vi "Compressor With Cylinder.vi"() -> ()   [LabVIEW 2014]
doc: "Compressor with Cylinder \n\nThis example shows how to control a compressor, extend and retract a cylinder, and optionally use a limit switch to retract automatically.\n\nThis example works with the PCM (Pneumatic Control Module) communicating with the roboRIO over CAN bus. The PCM must also be supplied with 12V DC from the PDP (Power Distribution Panel).\n\nThe Compressor, Pressure Switch, and Solenoids are all wired to the PCM \n\nThe Limit Switch is wired to DIO 9. It causes the cylinder to retract when the Auto Retract button is pressed.\n\nRefer to the Pneumatics Manual for air connections. Your pneumatics setup should include a compressor, pressure switch, tank, regulator, valve, flow controls, cylinder, plug valve, etc.\n\nTo run this example you should have a pneumatic system with air pressure connected to the P input on the SMC double solenoid valve. The A output of the valve should be connected via a flow control to the backend of a cylinder. The B output of the valve should be connected via a flow control to the frontend of a cylinder. When the cylinder is extended, it should physically depress the Limit Switch.\n\nWith the VI running, pressing the Extend button will push the cylinder shaft out, and pressing the Retract button will pull it back. Notice that the Extend and Retract buttons have their Mechanical Action set to Latch When Pressed. This means they stay pressed (ON) until they are read by the program, then they return to the OFF position. This works because once the SMC solenoid valve is pulled one direction, it stays in that position until it is pulled in the opposite direction - it only needs to be momentarily energized. The Auto Retract button can be used to make the cylinder return automatically. With the Auto Retract button ON, pressing the Extend button will push the cylinder out, and it will retract when it hits the limit switch.\n\nThis example expects a USB cable connected from your development PC to the Type B USB Jack (next to the power input) on the roboRIO.\n\nThis example expects the Driver Station to be running."
uses:
  <vilib>/Rock Robotics/WPI/Solenoid/WPI_SolenoidChannel.ctl
  <vilib>/Rock Robotics/SystemInterfaces/DIO/FPGA_DIOChannel.ctl
  <vilib>/Rock Robotics/WPI/Solenoid/WPI_SolenoidValue.ctl
  <vilib>/Rock Robotics/WPI/Solenoid/WPI_SolenoidOpenDouble.vi
  <vilib>/Rock Robotics/WPI/Solenoid/WPI_SolenoidSetEnum.vi
panel:
  in  "Retract 2":bool
  in  "Extend 2":bool
  in  "Extend Solenoid Channel 2":T1=enum."Solenoid 1"
  in  "Retract Solenoid Channel 2":T1
  out "Compressor Running":bool
  out "Cylinder Limit":bool
  in  "Limit Switch Channel":T2=enum."DIO 9"
  in  "Auto Retract":bool
  in  "Retract":bool
  in  "Retract Solenoid Channel":T1
  in  "Extend Solenoid Channel":T1=enum."Solenoid 1"
  out "Compressor Monitoring":bool
  in  "stop":bool
  in  "Extend":bool
  # "Set these inputs before running."
  # "roboRIO Wiring Diagram"
  # "when extended, the cylinder should depress this"
  # "Limit\nSwitch"
  # "These can be set while running."
  # "Pneumatic Control Module Wiring Diagram"
  # "Output information."
  # "Connect\nPower in\nHere"
  # "Connect\nCompressor\nHere"
  # "tubing port for retract side of cylinder"
  # "tubing port for extend side of cylinder"
  # "Pressure\nSwitch"
  # "SMC double solenoid valve"
  # "CAN"
  # "COMPRESSOR OUT"
  # "PRESSURE"
  # "NC"
  # "C"
  # "B"
  # "A"
  # "B"
  # "A"
  # "COM"
  # "NC"
  # "NO"
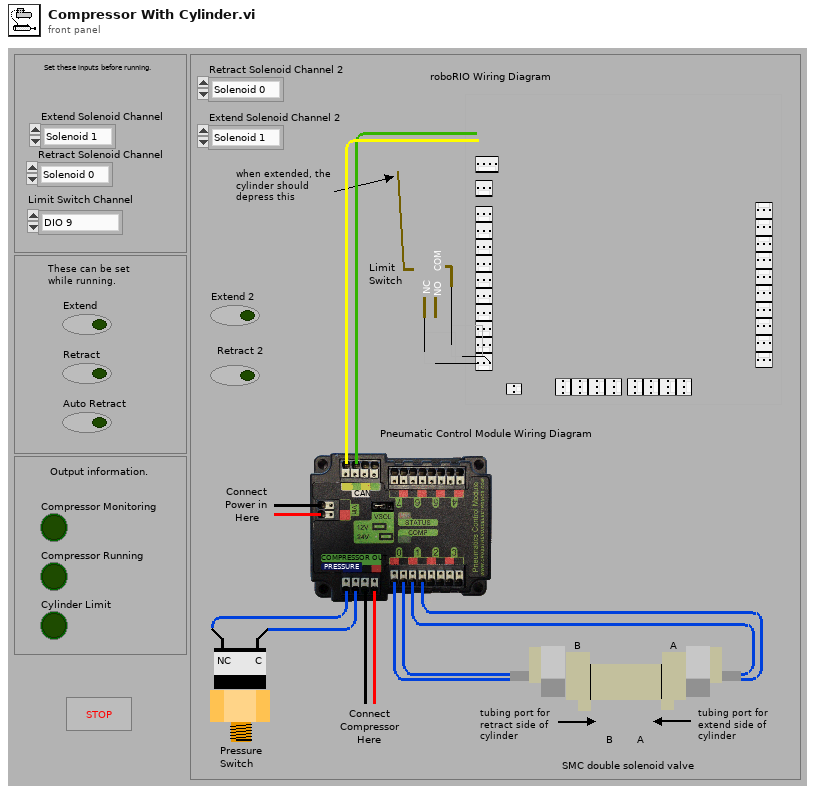
[diagram p1: front panel]
types:
  T1 = typedef "WPI_SolenoidChannel.ctl" = enum8{"Solenoid 0", "Solenoid 1", "Solenoid 2", "Solenoid 3", "Solenoid 4", "Solenoid 5", "Solenoid 6", "Solenoid 7", "Invalid"}
  T2 = typedef "FPGA_DIOChannel.ctl" = enum8{"DIO 0", "DIO 1", "DIO 2", "DIO 3", "DIO 4", "DIO 5", "DIO 6", "DIO 7", "DIO 8", "DIO 9", "DIO MXP 0", "DIO MXP 1", "DIO MXP 2", "DIO MXP 3", "DIO MXP 4", "DIO MXP 5", "DIO MXP 6", "DIO MXP 7", "DIO MXP 8", "DIO MXP 9", "DIO MXP 10", "DIO MXP 11", "DIO MXP 12", "DIO MXP 13", "DIO MXP 14", "DIO MXP 15", "Invalid"}
  T3 = typedef "WPI_CompressorDevRef.ctl" = cluster{"DevStatus":errorcluster, "Pneumatics Control Module":u8}
  T4 = typedef "WPI_SolenoidDevRef.ctl" = cluster{"DevStatus":errorcluster, "Pneumatics Control Module":u8, "Forward Solenoid Channel":T1, "Reverse Solenoid Channel":T1}
  T5 = typedef "WPI_DigitalInputDevRef.ctl" = cluster{"DevStatus":errorcluster, "DIO Channel":T2, "Controller":T6}
  T6 = typedef "FPGA_TypedefDigitalModule.ctl" = enum16{"Controller 1"}
  T7 = typedef "WPI_SolenoidValue.ctl" = enum16{"Off", "On", "Forward", "Reverse"}
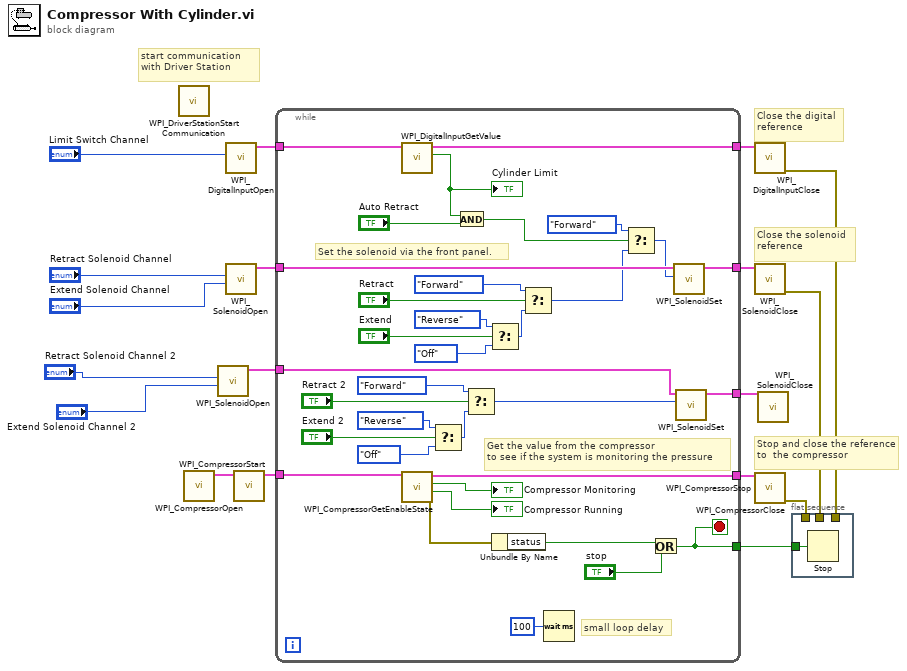
[diagram p0: block diagram]
diagram:
  # "Close the digital\nreference"
  # "Close the solenoid\nreference"
  # "start communication with Driver Station"
  # "Stop and close the reference to  the compressor"
  n1 = call <vilib>:"WPI_DriverStationStart Communication.vi"() -> ()  [unwired: 2 in, 10 out]
  n2 = call <vilib>:"WPI_CompressorOpen.vi"() -> ("CompressorDevRef"=w9:T3)  [unwired: 14 in, 1 out]
  n3 = call-poly <vilib>:"WPI_SolenoidOpen.vi"("Reverse Solenoid Channel"="Extend Solenoid Channel 2", "Forward Solenoid Channel"="Retract Solenoid Channel 2") -> ("SolenoidDevRef"=w3:T4)  [unwired: 2 in, 7 out]
  n4 = call <vilib>:"WPI_DigitalInputOpen.vi"("DIO Channel"="Limit Switch Channel") -> ("DigitalInputDevRef"=w13:T5)  [unwired: 2 in, 8 out]
  n5 = call-poly <vilib>:"WPI_SolenoidOpen.vi"("Reverse Solenoid Channel"="Extend Solenoid Channel", "Forward Solenoid Channel"="Retract Solenoid Channel") -> ("SolenoidDevRef"=w15:T4)  [unwired: 2 in, 7 out]
  n6 = call <vilib>:"WPI_CompressorStart.vi"("CompressorDevRef"=w9) -> ("CompressorDevRef"=w18:T3)  [unwired: 1 in, 9 out]
  n7 = while {
    tunnel: w18 -> [w53]
    tunnel: [w52] -> w17
    tunnel: [w50] -> w8
    tunnel: w15 -> [w45]
    tunnel: [w35] -> w16
    tunnel: w13 -> [w44]
    tunnel: [w43] -> w12
    tunnel: [w28] -> w4
    tunnel: w3 -> [w27]
    stop <- w50 stop-if-true
    # "small loop delay"
    # "Get the value from the compressor \nto see if the system is monitoring the pressure"
    # "Set the solenoid via the front panel."
    n8 = call <vilib>:"WPI_DigitalInputGetValue.vi"("DigitalInputDevRef"=w44) -> ("Value"=w33:bool, "DigitalInputDevRef"=w43:T5)  [unwired: 1 in, 8 out]
    "Cylinder Limit" <- w33
    n9 = call <vilib>:"WPI_CompressorGetEnableState.vi"("CompressorDevRef"=w53) -> ("error out"=w48:errorcluster, "Compressor Running"=→"Compressor Running":bool, "Enabled"=→"Compressor Monitoring":bool, "CompressorDevRef"=w52:T3)  [unwired: 1 in, 6 out]
    n10 = Select(t=WPI_SolenoidValue."Reverse" ("Value"), s="Extend 2", f=WPI_SolenoidValue."Off" ("Value")) -> (s? t:f=w22:T7)
    n11 = And(x=w33, y="Auto Retract") -> (x .and. y?=w29:bool)
    n12 = Select(t=WPI_SolenoidValue."Forward" ("Value"), s="Retract 2", f=w22) -> (s? t:f=w20:T7)
    n13 = Select(t=WPI_SolenoidValue."Reverse" ("Value"), s="Extend", f=WPI_SolenoidValue."Off" ("Value")) -> (s? t:f=w37:T7)
    n14 = Unbundle By Name(w48) -> ("status"=w47:bool)
    n15 = Select(t=WPI_SolenoidValue."Forward" ("Value"), s="Retract", f=w37) -> (s? t:f=w30:T7)
    n16 = Wait (ms)(milliseconds to wait=u32 100) -> ()  [unwired: 1 out]
    n17 = Select(t=WPI_SolenoidValue."Forward" ("Value"), s=w29, f=w30) -> (s? t:f=w31:T7)
    n18 = Or(x=w47, y="stop") -> (x .or. y?=w50:bool)
    n19 = call-poly <vilib>:"WPI_SolenoidSet.vi"("Value"=w31, "SolenoidDevRef"=w45) -> ("SolenoidDevRef"=w35:T4)  [unwired: 1 in, 8 out]
    n20 = call-poly <vilib>:"WPI_SolenoidSet.vi"("Value"=w20, "SolenoidDevRef"=w27) -> ("SolenoidDevRef"=w28:T4)  [unwired: 1 in, 8 out]
  }
  n21 = call <vilib>:"WPI_DigitalInputClose.vi"("DigitalInputDevRef"=w12) -> ("error out"=w5:errorcluster)  [unwired: 1 in, 9 out]
  n22 = call <vilib>:"WPI_SolenoidClose.vi"("SolenoidDevRef"=w16) -> ("error out"=w6:errorcluster)  [unwired: 1 in, 9 out]
  n23 = call <vilib>:"WPI_CompressorStop.vi"("CompressorDevRef"=w17) -> ("CompressorDevRef"=w19:T3)  [unwired: 1 in, 9 out]
  n24 = call <vilib>:"WPI_CompressorClose.vi"("CompressorDevRef"=w19) -> ("error out"=w7:errorcluster)  [unwired: 1 in, 9 out]
  n25 = call <vilib>:"WPI_SolenoidClose.vi"("SolenoidDevRef"=w4) -> ()  [unwired: 1 in, 10 out]
  n26 = flat-sequence {
    tunnel: w8 -> [w54]
    tunnel: w7 -> [_]
    tunnel: w6 -> [_]
    tunnel: w5 -> [_]
    frame #0 {
      n27 = Stop(stop? (T)=w54) -> ()
    }
  }
